vi "Configure List Sequence Repeat.vi"(8 "error in (no error)":errorcluster, 9 "Repeat Count (1)":i32=1 min=1 max=65535 step=1, 10 "Sequence Number (1)":i32=1 min=1 max=10 step=1 format="%#.0f", 11 "VISA resource name":refnum<visa-resource-name>) -> (0 "error out":errorcluster, 3 "VISA resource name out":refnum<visa-resource-name>)   [LabVIEW 2022 SP3]
doc: "Configures the repeat count of a selected sequence within list program. The selected sequence must be one of the linked sequences as configured in <b>Configure List Parameters.vi</b>, thus this vi should be run after <b>Configure List Parameters.vi</b>. Additionally, for all linked sequences configured in <b>Configure List Parameters.vi</b>, this vi must be used to configure each of those sequences' repeat count prior to saving the list program. For example, if sequence 2, 4, and 5 are selected linked sequences, then this vi must run afterwards to configure the repeat count for sequence 2, 4, and 5 subsequently."
uses:
  <instrlib>/BK Precision 911X Series/BK Precision 911X Series.lvlib
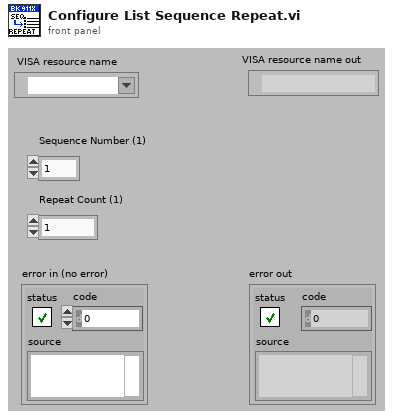
[diagram p1: front panel]
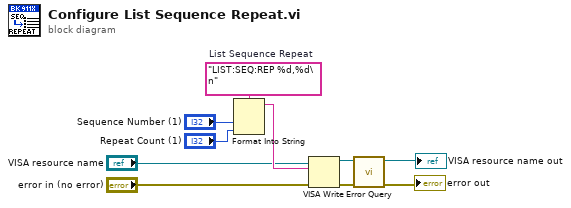
[diagram p0: block diagram]
diagram:
  w6 = "LIST:SEQ:REP %d,%d\n"  # List Sequence Repeat
  n1 = Format Into String(format string=w6, "Sequence Number (1)", "Repeat Count (1)") -> (resulting string=w5:string)  [unwired: 2 in, 1 out]
  n2 = VISA Write(VISA resource name="VISA resource name", write buffer=w5, error in (no error)="error in (no error)") -> (VISA resource name out=w10:refnum<visa-resource-name>, error out=w9:errorcluster)  [unwired: 1 out]
  n3 = call <instrlib>:"Error Query.vi"("error in (no error)"=w9, "VISA resource name"=w10) -> ("error out"=→"error out":errorcluster, "VISA resource name out"=→"VISA resource name out":refnum<visa-resource-name>)  [unwired: 6 in, 2 out]
